vi "Gyro_Example.vi"() -> ()   [LabVIEW 2019]
uses:
  <vilib>/Platform/TimedLoop/XDataNode/timing_clust.ctl
  <vilib>/Platform/TimedLoop/XDataNode/nitl_modes.ctl
  <vilib>/Platform/TimedLoop/XDataNode/wakeup.ctl
  <vilib>/myRIO/Instrument Drivers/Onboard IO/I2C/typedefs/I2C User Configuration.ctl
  <vilib>/myRIO/Instrument Drivers/Onboard IO/I2C/typedefs/I2C Transfer Rate.ctl
  <vilib>/myRIO/Instrument Drivers/Onboard IO/I2C/typedefs/I2C Reference.ctl
  <vilib>/myRIO/Common/Instrument Driver Framework/Utilities/typedefs/myRIO Generic Hardware Reference.ctl
  <vilib>/myRIO/Common/Instrument Driver Framework/Utilities/typedefs/Hardware Version Enum.ctl
  <vilib>/myRIO/Common/Instrument Driver Framework/Utilities/typedefs/myRIO v1.0 Reference.ctl
  <vilib>/myRIO/Common/Instrument Driver Framework/Utilities/typedefs/Generic FPGA Reference.ctl
  <vilib>/myRIO/Common/Instrument Driver Framework/myRIO v1.0/I2C/typedefs/I2C Channels Enum.ctl
  <vilib>/myRIO/Instrument Drivers/Onboard IO/I2C/typedefs/I2C Configuration.ctl
  <vilib>/userDefined/High Color/nirio_resource_hc.ctl
  <vilib>/myRIO/Common/Instrument Driver Framework/Utilities/vis/Is FPGA Ref Available.vi
  <vilib>/myRIO/Common/Instrument Driver Framework/myRIO v1.0/I2C/vis/myRIO v1.1 Open I2C.vi
  <vilib>/myRIO/Instrument Drivers/Onboard IO/I2C/vis/Configure.vi
  <vilib>/myRIO/Instrument Drivers/Onboard IO/I2C/vis/Write.vi
  <vilib>/myRIO/Instrument Drivers/Onboard IO/I2C/vis/Write Read.vi
  <vilib>/myRIO/Common/Instrument Driver Framework/Utilities/vis/Validate Channels.vi
  <vilib>/myRIO/Common/Instrument Driver Framework/myRIO v1.0/I2C/vis/myRIO v1.0 Reserve I2C.vi
  <vilib>/myRIO/Common/Instrument Driver Framework/myRIO v1.0/I2C/vis/myRIO v1.0 Build MUX Configuration I2C.vi
  <vilib>/myRIO/Common/Instrument Driver Framework/myRIO v1.0/Resource Manager/vis/myRIO v1.0 Reserve Channel List.vi
  <vilib>/myRIO/Common/Instrument Driver Framework/myRIO v1.0/Resource Manager/vis/myRIO v1.0 Create Configuration List.vi
  <vilib>/myRIO/Common/Instrument Driver Framework/myRIO v1.0/Resource Manager/vis/myRIO v1.0 Reserve Channel.vi
  <vilib>/myRIO/Common/Instrument Driver Framework/myRIO v1.0/Resource Manager/vis/myRIO v1.0 Unreserve Channel.vi
  <vilib>/myRIO/Common/Instrument Driver Framework/myRIO v1.0/Resource Manager/vis/myRIO v1.0 Build Mutex Name.vi
  <vilib>/Utility/VariantDataType/GetNumericInfo.vi
  <vilib>/Utility/error.llb/Error Cluster From Error Code.vi
  <vilib>/myRIO/Common/Instrument Driver Framework/myRIO v1.0/myRIO v1.1 Open.vi
  <vilib>/myRIO/Common/Instrument Driver Framework/Utilities/vis/IO Manager.vi
  <vilib>/myRIO/Common/Instrument Driver Framework/Utilities/vis/Configuration Manager.vi
  <vilib>/myRIO/Common/Instrument Driver Framework/myRIO v1.0/Resource Manager/vis/myRIO v1.0 Configure IO.vi
  <vilib>/myRIO/Common/Instrument Driver Framework/myRIO v1.0/myRIO v1.0 Close.vi
  <vilib>/myRIO/Common/Instrument Driver Framework/myRIO v1.0/I2C/vis/myRIO v1.0 Configure I2C.vi
  <vilib>/myRIO/Common/Instrument Driver Framework/myRIO v1.0/I2C/vis/myRIO v1.0 Write I2C.vi
  <vilib>/myRIO/Common/Instrument Driver Framework/myRIO v1.0/I2C/vis/myRIO v1.0 Read I2C.vi
  <vilib>/myRIO/Express VI/Onboard IO/I2C/I2C Express VI.xnode
  <vilib>/myRIO/Instrument Drivers/Onboard IO/I2C/vis/myRIO I2C Open.xnode
  <vilib>/platform/TimedLoop/XDataNode/XDataNode.xnode
  <vilib>/myRIO/Instrument Drivers/Onboard IO/I2C/I2C.lvlib
  <vilib>/Platform/TimedLoop/XDataNode/XDNodeRunTimeDep.lvlib
  <vilib>/ptbypt/NI_PtbyPt.lvlib
panel:
  out "error out 3":errorcluster
  out "error out 2":errorcluster
  out "Array":u8[](array[numeric])
  out "error out":errorcluster
  in  "Reset":bool
  out "Finished Late? [i-1]":bool
  out "Bytes Read":u8[](array[numeric]) format="%.0x"
  in  "Stop Button 2":bool
  out "x/y 2":dbl[](array[numeric])
  out "x/y":dbl[](array[numeric])
  out "mean":dbl format="%0.2f"
  out "Finished Late? [i-1] 2":bool
  in  "Stop Button":bool
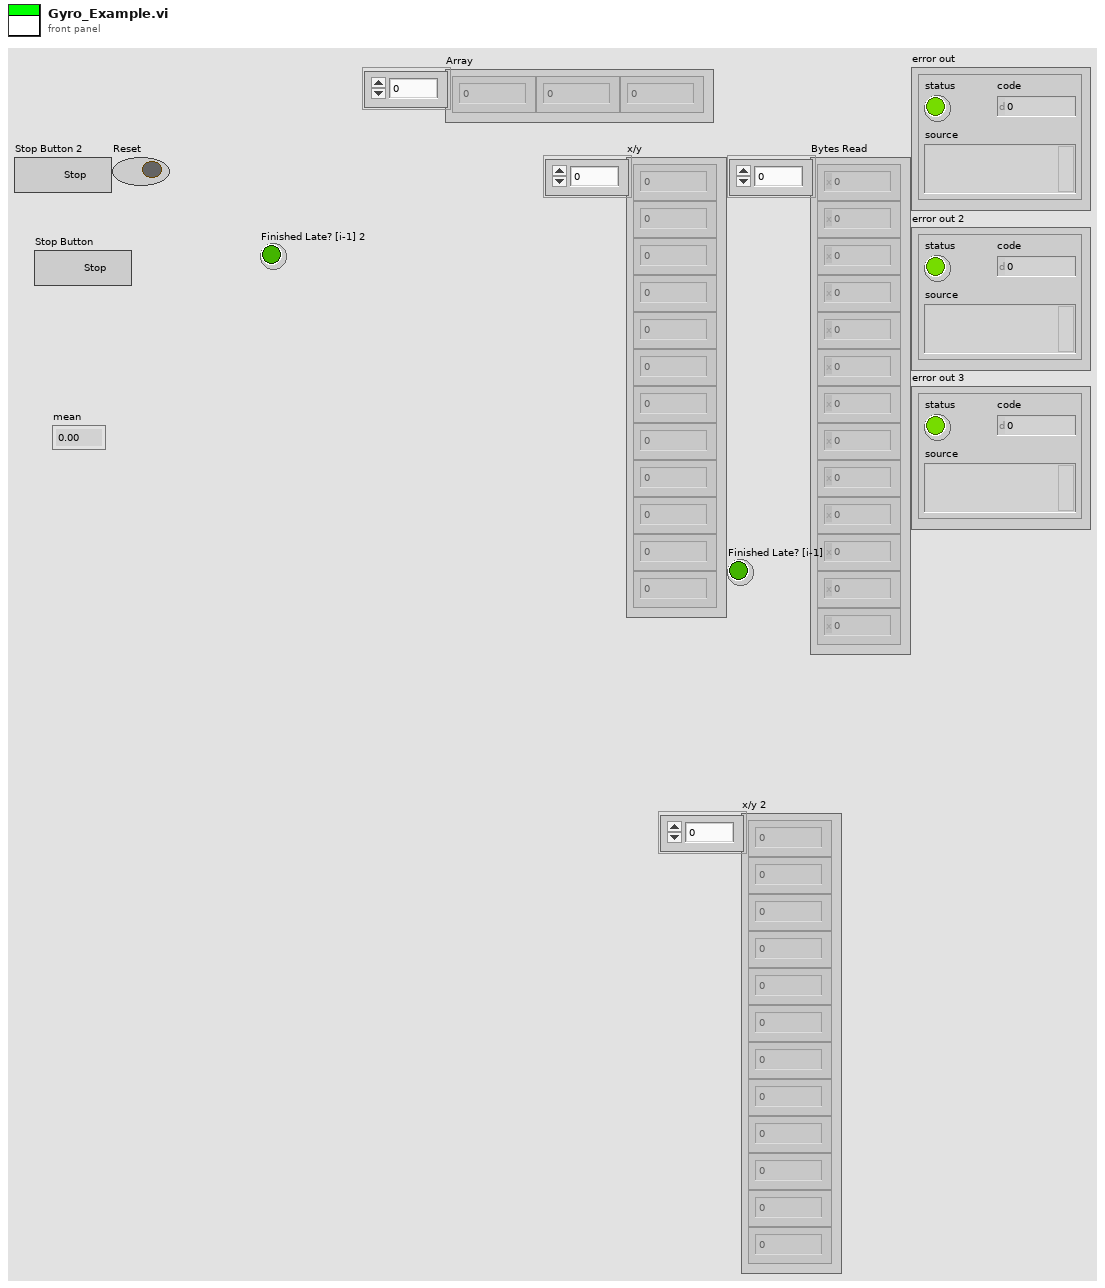
[diagram p1: front panel]
types:
  T1 = typedef "I2C.lvlib/I2C Reference.ctl" = cluster{"myRIO Reference":T2, "I2C Channels Enum":T6, "I2C Configuration":T7}
  T2 = typedef "myRIO Generic Hardware Reference.ctl" = cluster{"myRIO Model":T3, "myRIO Hardware Reference":T4}
  T3 = typedef "Hardware Version Enum.ctl" = enum16{"Unknown", "myRIO-1900", "myRIO-1950", "roboRIO", "NI ELVIS RIO CM", "ELVIS III"}
  T4 = typedef "myRIO v1.0 Reference.ctl" = cluster{"Generic FPGA Reference":T5, "Allow multiple opens":bool}
  T5 = typedef "Generic FPGA Reference.ctl" = refnum<k20>
  T6 = typedef "I2C Channels Enum.ctl" = enum16{"Not Connected", "A/I2C", "B/I2C", "I2C/I2C"}
  T7 = typedef "I2C.lvlib/I2C Configuration.ctl" = cluster{"I2C Transfer Rate":T8}
  T8 = typedef "I2C.lvlib/I2C Transfer Rate.ctl" = enum16{"Standard mode (100 kbps)", "Fast mode (400 kbps)"}
  T9 = typedef "I2C.lvlib/I2C User Configuration.ctl" = cluster{"I2C Transfer Rate":T8}
  T10 = typedef "nirio_resource_hc.ctl" = tag
  T11 = typedef "XDNodeRunTimeDep.lvlib/timing_clust.ctl" = cluster{"Expected End [f-1]":u64, "Actual End [f-1]":u64, "Finished Late? [f-1]":bool, "Expected End [i-1]":u64, "Actual End [i-1]":u64, "Finished Late? [i-1]":bool, "Expected Start [i]":u64, "Actual Start [i]":u64, "Expected Start [f]":u64, "Actual Start [f]":u64, "Source Name":string, "Structure Name":string, "Period":i64, "Deadline":i64, "Offset":i64, "Start":i64, "Priority":i32, "Timeout":i32, "Mode":T12, "Wakeup Reason":T13, "Error":errorcluster, "Source Type":string, "Secondary Source Type":string, "Global End Time":u64, "Global Start Time":u64, "Frame Duration":u64, "Iteration Duration":u64, "Assigned CPU":i32, "I/O Scan Engine Mode":u32}
  T12 = typedef "XDNodeRunTimeDep.lvlib/nitl_modes.ctl" = enum32{"No Change", "Process missed periods, maintain original phase", "Discard missed periods, maintain original phase", "Process missed periods, ignore original phase", "Discard missed periods, ignore original phase"}
  T13 = typedef "XDNodeRunTimeDep.lvlib/wakeup.ctl" = enum32{"Normal", "Aborted", "Asynchronous wakeup", "Timing source error", "Timed loop error", "Timeout"}
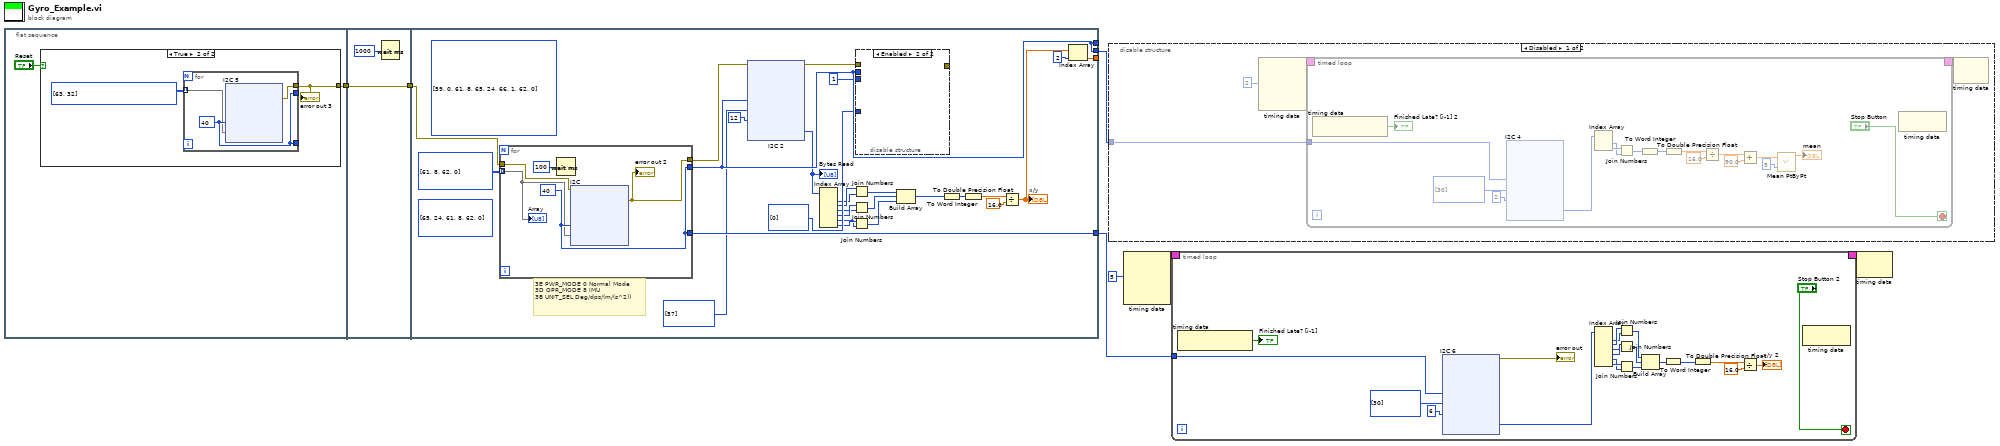
[diagram p0: block diagram]
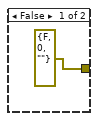
[diagram p3: hidden frame]
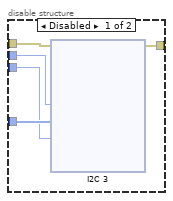
[diagram p4: hidden frame]
diagram:
  n1 = flat-sequence {
    tunnel: [w9] -> w1
    tunnel: [w54] -> w2
    tunnel: w1 -> [w54]
    tunnel: [w80] -> w7
    tunnel: [w79] -> w4
    tunnel: [w81] -> _
    tunnel: [w80] -> _
    tunnel: w2 -> [w57]
    frame #0 {
      n2 = case shown="True" "Reset" {
        tunnel: [errorcluster {"status"=FALSE, "code"=0, "source"=""} ("error out") w11] -> w9
        frame False {
        }
        frame True {
          n3 = for {
            tunnel: [w15] -> w11
            tunnel: [w14] -> _
            tunnel: [w14] -> _
            tunnel: u8[][] [[63, 32]] ("Bytes to Write") -> [w13] mode=indexing
            w14 = u8 40 ("Slave Address (7-bit)")
            n4 = xnode "I2C 5"("Slave Address (7-bit)"=w14, "Bytes to Write"=w13) -> ("error out"=w15:errorcluster)  [unwired: 1 in]
          }
          "error out 3" <- w11
        }
      }
    }
    frame #1 {
      n5 = Wait (ms)(milliseconds to wait=u32 1000) -> ()  [unwired: 1 out]
    }
    frame #2 {
      (unwired) u8[][] [[65, 24], [61, 8], [62, 0]]
      (unwired) u8[][] [[59, 0], [61, 8], [65, 24], [66, 1], [62, 0]] ("Bytes to Write")
      # "3E PWR_MODE 0 Normal Mode\n3D OPR_MODE 8 IMU\n3B UNIT_SEL Deg/dps/(m/(s^2))"
      n6 = for {
        tunnel: [w172] -> w82
        tunnel: [w171] -> w80
        tunnel: u8[][] [[61, 8], [62, 0]] -> [w170] mode=indexing
        tunnel: [w171] -> w79
        tunnel: w57 -> [w168]
        w171 = u8 40 ("Slave Address (7-bit)")
        n7 = Wait (ms)(milliseconds to wait=u32 100) -> ()  [unwired: 1 out]
        n8 = xnode "I2C"("Slave Address (7-bit)"=w171, "Bytes to Write"=w170, "error in (no error)"=w168) -> ("error out"=w172:errorcluster)
        "error out 2" <- w172
        "Array" <- w170
      }
      n9 = xnode "I2C 2"("Slave Address (7-bit)"=w80, "Bytes to Write"=u8[] [57], "Byte Count"=u32 12, "error in (no error)"=w82) -> ("Bytes Read"=w73:u8[], "error out"=w76:errorcluster)
      "Bytes Read" <- w73
      n10 = Index Array(array=w73) -> (element #1=w71:u8, element #2=w72:u8, element #3=w60:u8, element #4=w61:u8, element #5=w69:u8, element #6=w70:u8)  [unwired: 6 in]
      n11 = Join Numbers(hi=w72, lo=w71) -> ((hi.lo)=w68:u16)
      n12 = Join Numbers(hi=w61, lo=w60) -> ((hi.lo)=w67:u16)
      n13 = Join Numbers(hi=w70, lo=w69) -> ((hi.lo)=w66:u16)
      n14 = disable-structure shown="Enabled" {
        disable-tunnel: w76 -> [w87 _]
        disable-tunnel: u8[] [0] ("Bytes to Write") -> [w86 _]
        disable-tunnel: u32 1 ("Byte Count") -> [w85 _]
        disable-tunnel: [w84 _] -> _
        disable-tunnel: w80 -> [w83 _]
        frame Disabled {
          n15 = xnode "I2C 3"("Slave Address (7-bit)"=w83, "Bytes to Write"=w86, "Byte Count"=w85, "error in (no error)"=w87) -> ("error out"=w84:errorcluster)  [unwired: 1 out]
        }
        frame Enabled {
        }
      }
      n16 = Build Array(w68, w67, w66) -> (w62:u16[])
      n17 = To Word Integer(number=w62) -> (16bit integer=w63:i16[])
      n18 = To Double Precision Float(number=w63) -> (double precision float=w65:dbl[])
      n19 = Divide(x=w65, y=16.0) -> (x/y=w59:dbl[])
      "x/y" <- w59
      n20 = Index Array(array=w59, index=2) -> (element=w81:dbl)
    }
  }
  n21 = disable-structure shown="Disabled" {
    disable-tunnel: w7 -> [w212 _]
    frame Disabled {
      n22 = node-c288(i64 2 ("Period")) -> (w214:T11)  [unwired: 3 in]
      n23 = timed-loop {
        timing: w214 -> [_]
        timing-out: [_] -> w213
        tunnel: w212 -> [w220]
        stop <- "Stop Button" stop-if-true
        n24 = node-c288() -> (→"Finished Late? [i-1] 2":bool)  [unwired: 1 in]
        n25 = xnode "I2C 4"("Slave Address (7-bit)"=w220, "Bytes to Write"=u8[] [30], "Byte Count"=u32 2) -> ("Bytes Read"=w221:u8[])  [unwired: 1 in, 1 out]
        n26 = Index Array(array=w221) -> (element #1=w228:u8, element #2=w229:u8)  [unwired: 2 in]
        n27 = Join Numbers(hi=w229, lo=w228) -> ((hi.lo)=w227:u16)
        n28 = To Word Integer(number=w227) -> (16bit integer=w226:i16)
        n29 = To Double Precision Float(number=w226) -> (double precision float=w225:dbl)
        n30 = Divide(x=w225, y=16.0) -> (x/y=w223:dbl)
        n31 = Add(x=w223, y=90.0) -> (x+y=w218:dbl)
        n32 = call <vilib>:"Mean PtByPt.vi"("x"=w218, "sample length"=5) -> ("mean"=→"mean":dbl)  [unwired: 2 in, 1 out]
        n33 = node-c288() -> ()  [unwired: 1 in, 1 out]
      }
      n34 = node-c288(w213) -> ()  [unwired: 1 out]
    }
    frame Enabled {
    }
  }
  n35 = node-c288(i64 5 ("Period")) -> (w6:T11)  [unwired: 3 in]
  n36 = timed-loop {
    timing: w6 -> [_]
    timing-out: [_] -> w5
    tunnel: w4 -> [w282]
    stop <- "Stop Button 2" stop-if-true
    n37 = node-c288() -> (→"Finished Late? [i-1]":bool)  [unwired: 1 in]
    n38 = xnode "I2C 6"("Slave Address (7-bit)"=w282, "Bytes to Write"=u8[] [30], "Byte Count"=u32 6) -> ("Bytes Read"=w297:u8[], "error out"=→"error out":errorcluster)  [unwired: 1 in]
    n39 = Index Array(array=w297) -> (element #1=w295:u8, element #2=w296:u8, element #3=w284:u8, element #4=w285:u8, element #5=w293:u8, element #6=w294:u8)  [unwired: 6 in]
    n40 = Join Numbers(hi=w296, lo=w295) -> ((hi.lo)=w292:u16)
    n41 = Join Numbers(hi=w285, lo=w284) -> ((hi.lo)=w291:u16)
    n42 = Join Numbers(hi=w294, lo=w293) -> ((hi.lo)=w290:u16)
    n43 = Build Array(w292, w291, w290) -> (w286:u16[])
    n44 = To Word Integer(number=w286) -> (16bit integer=w287:i16[])
    n45 = To Double Precision Float(number=w287) -> (double precision float=w289:dbl[])
    n46 = Divide(x=w289, y=16.0) -> (x/y=→"x/y 2":dbl[])
    n47 = node-c288() -> ()  [unwired: 1 in, 1 out]
  }
  n48 = node-c288(w5) -> ()  [unwired: 1 out]
